vi "SVL Single Block Integration (1 Ch).vi"(7 "length units":i32(ring) items=["no change"=-1, "m"=0, "mm"=2, "microns"=3, "in"=1, "mils"=5], 8 "error in (no error)":errorcluster, 9 "known condition":T1={"condition type"=enum."Initial Value", "known value"=nan}, 11 "scaled signal [EU]":waveform(dbl)={"t0"=timestamp(0 s since 1904-01-01), "dt"=1.0, "Y"=[0.0]}) -> (0 "error out":errorcluster, 2 "unit label":string, 3 "integrated signal [EU*s]":waveform(dbl)={"t0"=timestamp(0 s since 1904-01-01), "dt"=1.0, "Y"=[], "attributes"=variant("NI_SV_ChannelInfo"=variant(cluster{"sensor sensitivity [mV/EU]":dbl, "engineering units":enum16{"custom...", "V", "Pa", "g", "m/s^2", "m/s", "m", "in/s^2", "in/s", "in"}, "dB reference [EU]":dbl, "custom label":string, "weighting filter":enum16{"Linear", "A-weighting", "B-weighting", "C-weighting"}, "pregain [dB]":dbl} {"sensor sensitivity [mV/EU]"=1000.0, "engineering units"=enum."custom...", "dB reference [EU]"=1.0, "custom label"="not found*s^2", "weighting filter"=enum."Linear", "pregain [dB]"=0.0}))})   [LabVIEW 2017, in "SoundVib_Integration.lvlib"]
doc: "Converts acceleration to velocity or displacement using a time-domain waveform as the input. Wire data to the <B>scaled signal [EU]</B> input to determine the polymorphic instance to use or manually select the instance.\n\nIntegrates a single block of data. Use this VI to numerically integrate a single block of data. Use the known condition input to correct the integrated signal for that known condition. The <B>condition type</B> value of the <B>known condition</B> input determines how the intergrated signal is adjusted, and the <B>known value</B> determines by how much it is adjusted. <B>condition type</B> can be <B>Initial Value</B>, <B>Mean Value</B>, or <B>Final Value</B>. Using <B>Initial Value</B> will offset the integrated signal so that the first value is eqaul to the known value. Using <B>Mean Value</B> will offset the integrated signal so that its mean is eqaul to the known value. And finally, using <B>Final Value</B> will offset the integrated signal so that its last value is eqaul to the known value. If <B>known value</B> is set to NaN, no adjustment will be performed (this is the default if unwired)."
uses:
  <vilib>/addons/Sound and Vibration/svt_Integration/SoundVib_Integration.lvlib
  <vilib>/addons/_NISVFA/_Shared subVIs/Controls/svc_Integration Known Condition.ctl
  <vilib>/Analysis/2dsp.llb/Integral x(t).vi
  <vilib>/Analysis/baseanly.llb/Mean.vi
  <vilib>/Analysis/baseanly.llb/Mean (DBL).vi
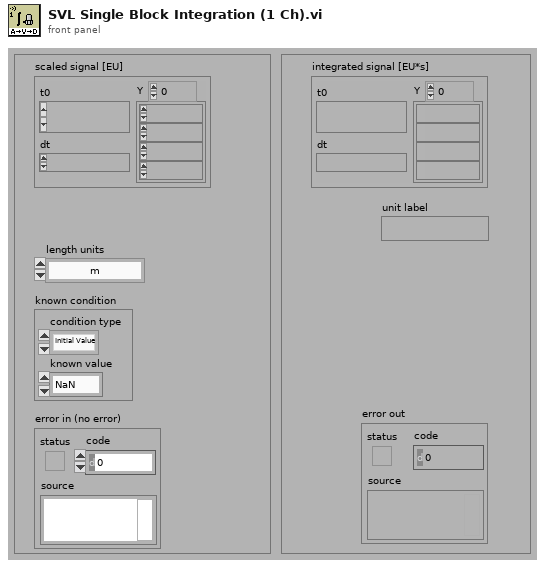
[diagram p1: front panel]
types:
  T1 = typedef "svc_Integration Known Condition.ctl" = cluster{"condition type":enum16{"Initial Value", "Mean Value", "Final Value"}, "known value":dbl}
  T2 = enum16{"single integration", "double integration"}
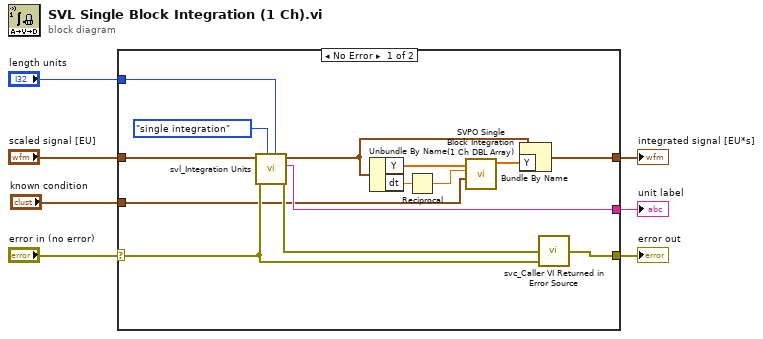
[diagram p0: block diagram]
diagram:
  n1 = case shown="No Error" "error in (no error)" {
    selector: "error in (no error)" -> [w18 w22]
    tunnel: "scaled signal [EU]" -> [w10 _]
    tunnel: [w8 _] -> w6
    tunnel: [w21 w22] -> w5
    tunnel: [w19 _] -> w4
    tunnel: "length units" -> [w20 _]
    tunnel: "known condition" -> [w12 _]
    frame No Error {
      n2 = call <vilib>:"svl_Integration Units.vi"("desired base units for length"=w20, "integration type"=T2."single integration", "error in (no error)"=w18, "scaled signal [EU]"=w10) -> ("error out"=w17:errorcluster, "unit label"=w19:string, "scaled signal out"=w9:waveform(dbl))  [unwired: 5 in]
      n3 = Unbundle By Name(w9) -> ("Y"=w15:dbl[], "dt"=w14:dbl)
      n4 = Reciprocal(x=w14) -> (1/x=w13:dbl)
      n5 = call <vilib>:"SVPO Single Block Integration (1 Ch DBL Array).vi"("known condition"=w12, "sampling rate [Hz]"=w13, "scaled signal [EU]"=w15) -> ("integrated signal [EU*s]"=w11:dbl[])  [unwired: 8 in]
      n6 = Bundle By Name(cluster=w9, "Y"=w11) -> (w8:waveform(dbl))
      n7 = call <vilib>:"svc_Caller VI Returned in Error Source.vi"("warning input to caller"=w18, "error in (no error)"=w17) -> ("error out"=w21:errorcluster)  [unwired: 3 in]
    }
    frame Error {
    }
  }
  "integrated signal [EU*s]" <- w6
  "error out" <- w5
  "unit label" <- w4
